vi "Configure Voltage Slew Rate.vi"(0 "VISA resource name":refnum<visa-resource-name>, 5 "Voltage Slew Rate Mode (0: Fixed)":i32(ring) items=["Fixed", "Step", "Pulse", "List"], 7 "Voltage Slew Rate (1e-3 Hz)":dbl=0.001, 9 "Triggered Voltage Slew Rate (1e-3 Hz)":dbl=0.001, 11 "error in (no error)":errorcluster) -> (4 "VISA resource name out":refnum<visa-resource-name>, 15 "error out":errorcluster)   [LabVIEW 2013, in "California Instruments iX Series.lvlib"]
doc: "Configures the voltage slew rate mode, voltage slew rate and triggered voltage slew rate."
uses:
  California Instruments iX Series.lvlib
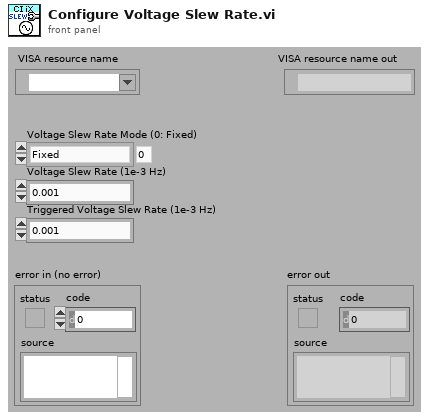
[diagram p1: front panel]
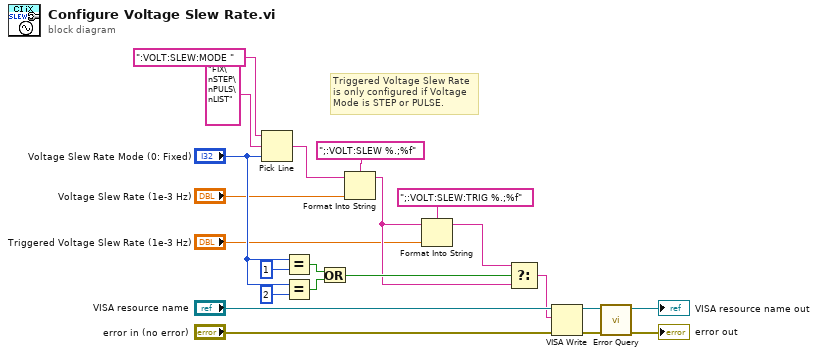
[diagram p0: block diagram]
diagram:
  # "Triggered Voltage Slew Rate is only configured if Voltage Mode is STEP or PULSE."
  n1 = Pick Line(string ("")=":VOLT:SLEW:MODE ", multi-line string="FIX\nSTEP\nPULS\nLIST", line index="Voltage Slew Rate Mode (0: Fixed)") -> (output string=w14:string)
  n2 = Equal?(x="Voltage Slew Rate Mode (0: Fixed)", y=1) -> (x = y?=w9:bool)
  n3 = Equal?(x="Voltage Slew Rate Mode (0: Fixed)", y=2) -> (x = y?=w8:bool)
  n4 = Or(x=w9, y=w8) -> (x .or. y?=w7:bool)
  n5 = Format Into String(format string=";:VOLT:SLEW %.;%f", initial string=w14, "Voltage Slew Rate (1e-3 Hz)") -> (resulting string=w6:string)  [unwired: 1 in, 1 out]
  n6 = Format Into String(format string=";:VOLT:SLEW:TRIG %.;%f", initial string=w6, "Triggered Voltage Slew Rate (1e-3 Hz)") -> (resulting string=w5:string)  [unwired: 1 in, 1 out]
  n7 = Select(t=w5, s=w7, f=w6) -> (s? t:f=w1:string)
  n8 = VISA Write(VISA resource name="VISA resource name", write buffer=w1, error in (no error)="error in (no error)") -> (VISA resource name out=w20:refnum<visa-resource-name>, error out=w19:errorcluster)  [unwired: 1 out]
  n9 = call "Error Query.vi"("error in (no error)"=w19, "VISA resource name"=w20) -> ("error out"=→"error out":errorcluster, "VISA resource name out"=→"VISA resource name out":refnum<visa-resource-name>)  [unwired: 6 in, 2 out]
